vi "initDB.vi"   [LabVIEW 2014]
uses:
  <vilib>/Rock Robotics/Network Tables/SD Write Boolean.vi
  <vilib>/Rock Robotics/Network Tables/SD Write Number.vi
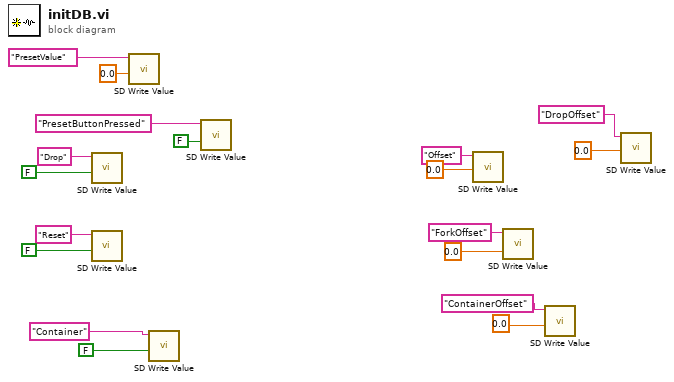
[diagram p0: block diagram]
diagram:
  n1 = call-poly <vilib>:"SD Write Value.vi"("Boolean"=FALSE, "Name"="Drop") -> ()  [unwired: 8 in, 2 out]
  n2 = call-poly <vilib>:"SD Write Value.vi"("Boolean"=FALSE, "Name"="Reset") -> ()  [unwired: 8 in, 2 out]
  n3 = call-poly <vilib>:"SD Write Value.vi"("Numeric"=0.0, "Name"="PresetValue") -> ()  [unwired: 8 in, 2 out]
  n4 = call-poly <vilib>:"SD Write Value.vi"("Boolean"=FALSE, "Name"="Container") -> ()  [unwired: 8 in, 2 out]
  n5 = call-poly <vilib>:"SD Write Value.vi"("Boolean"=FALSE, "Name"="PresetButtonPressed") -> ()  [unwired: 8 in, 2 out]
  n6 = call-poly <vilib>:"SD Write Value.vi"("Numeric"=0.0, "Name"="Offset") -> ()  [unwired: 8 in, 2 out]
  n7 = call-poly <vilib>:"SD Write Value.vi"("Numeric"=0.0, "Name"="ForkOffset") -> ()  [unwired: 8 in, 2 out]
  n8 = call-poly <vilib>:"SD Write Value.vi"("Numeric"=0.0, "Name"="ContainerOffset") -> ()  [unwired: 8 in, 2 out]
  n9 = call-poly <vilib>:"SD Write Value.vi"("Numeric"=0.0, "Name"="DropOffset") -> ()  [unwired: 8 in, 2 out]
